vi "make raise loop stop.vi"(8 "error in (no error)":errorcluster) -> (0 "error out":errorcluster)   [LabVIEW 2019]
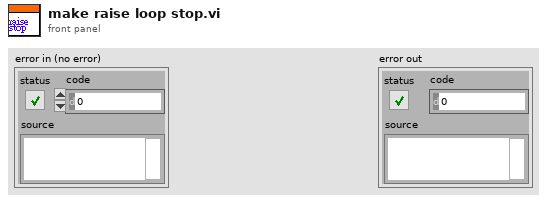
[diagram p1: front panel]
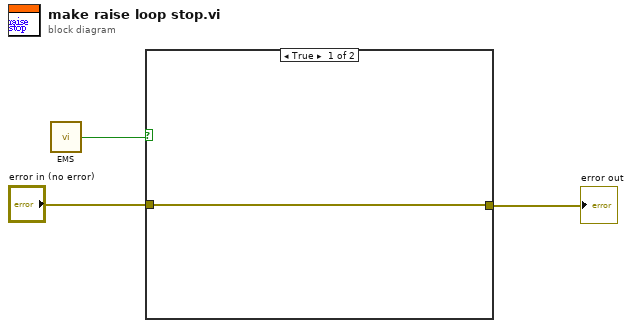
[diagram p0: block diagram]
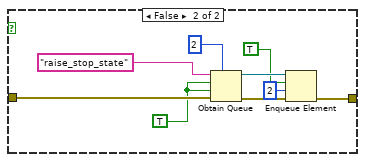
[diagram p2: hidden frame]
diagram:
  n1 = call "EMS.vi"() -> ("A/DIO4 (Pin 19)"=w1:bool)
  n2 = case shown="True" w1 {
    tunnel: "error in (no error)" -> [w4 w11]
    tunnel: [w4 w7] -> w2
    frame True {
    }
    frame False {
      w6 = TRUE
      n3 = Obtain Queue(max queue size (-1, unlimited)=2, name (unnamed)="raise_stop_state", element data type=w6, create if not found? (T)=w6, error in (no error)=w11) -> (queue out=w9:refnum<queue>, error out=w10:errorcluster)  [unwired: 1 out]
      n4 = Enqueue Element(queue=w9, element=TRUE, timeout in ms (-1)=2, error in (no error)=w10) -> (error out=w7:errorcluster)  [unwired: 2 out]
    }
  }
  "error out" <- w2
